vi "VideoPathBuilder.vi"(11 "Event Info":T1) -> (3 "Video Path":path)   [LabVIEW 2017]
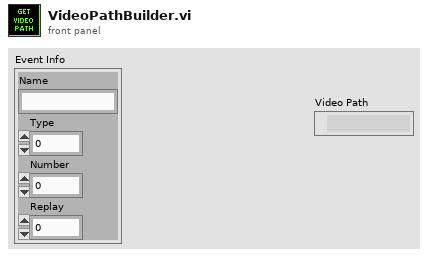
[diagram p1: front panel]
types:
  T1 = cluster{"Name":string, "Type":u8, "Number":u16, "Replay":u8}
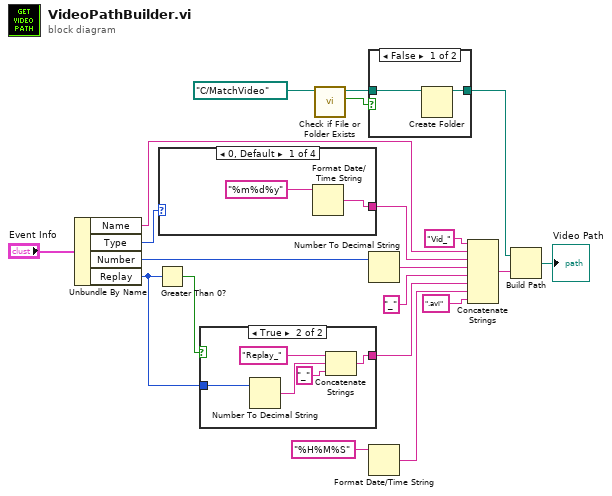
[diagram p0: block diagram]
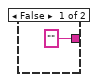
[diagram p3: hidden frame]
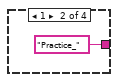
[diagram p4: hidden frame]
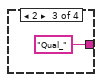
[diagram p5: hidden frame]
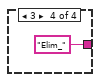
[diagram p6: hidden frame]
diagram:
  n1 = Unbundle By Name("Event Info") -> ("Name"=w5:string, "Type"=w3:u8, "Number"=w4:u16, "Replay"=w2:u8)
  n2 = Greater Than 0?(x=w2) -> (x > 0?=w18:bool)
  n3 = case shown="0, Default" w3 {
    tunnel: [w21 "Practice_" "Qual_" "Elim_"] -> w16
    frame 0, Default {
      n4 = Format Date/Time String(time format string (%c)="%m%d%y") -> (date/time string=w21:string)  [unwired: 2 in]
    }
    frame 1 {
    }
    frame 2 {
    }
    frame 3 {
    }
  }
  n5 = case shown="True" w18 {
    tunnel: w2 -> [_ w31]
    tunnel: ["" w27] -> w19
    frame False {
    }
    frame True {
      n6 = Number To Decimal String(number=w31) -> (decimal integer string=w29:string)  [unwired: 1 in]
      n7 = Concatenate Strings("Replay_" ("string"), w29, "_" ("string")) -> (w27:string)
    }
  }
  n8 = call <vilib>:"Check if File or Folder Exists.vi"("path"=path "C:/MatchVideo") -> ("file or folder exists?"=w12:bool, "dup path"=w11:path)  [unwired: 8 in, 1 out]
  n9 = case shown="False" w12 {
    tunnel: w11 -> [w33 w34]
    tunnel: [w32 w34] -> w10
    frame False {
      n10 = Create Folder(path (use dialog)=w33) -> (created path=w32:path)  [unwired: 2 in, 2 out]
    }
    frame True {
    }
  }
  n11 = Number To Decimal String(number=w4) -> (decimal integer string=w17:string)  [unwired: 1 in]
  n12 = Format Date/Time String(time format string (%c)="%H%M%S") -> (date/time string=w7:string)  [unwired: 2 in]
  n13 = Concatenate Strings("Vid_" ("string"), w5, w16, w17, "_" ("string"), w19, w7, ".avi" ("string")) -> (w20:string)
  n14 = Build Path(base path=w10, name or relative path=w20) -> (appended path=→"Video Path":path)
